vi "inputs_to_commands.vi"(11 "Joysticks":T6) -> (3 "Commands":T1)   [LabVIEW 2012]
uses:
  <vilib>/Rock Robotics/WPI/Joystick/WPI_JoystickButtonState.ctl
  Commands.ctl
  mecanum/mecanum_control.ctl
  Shooter/shooter_cmds.ctl
  climber/climber_cmds.ctl
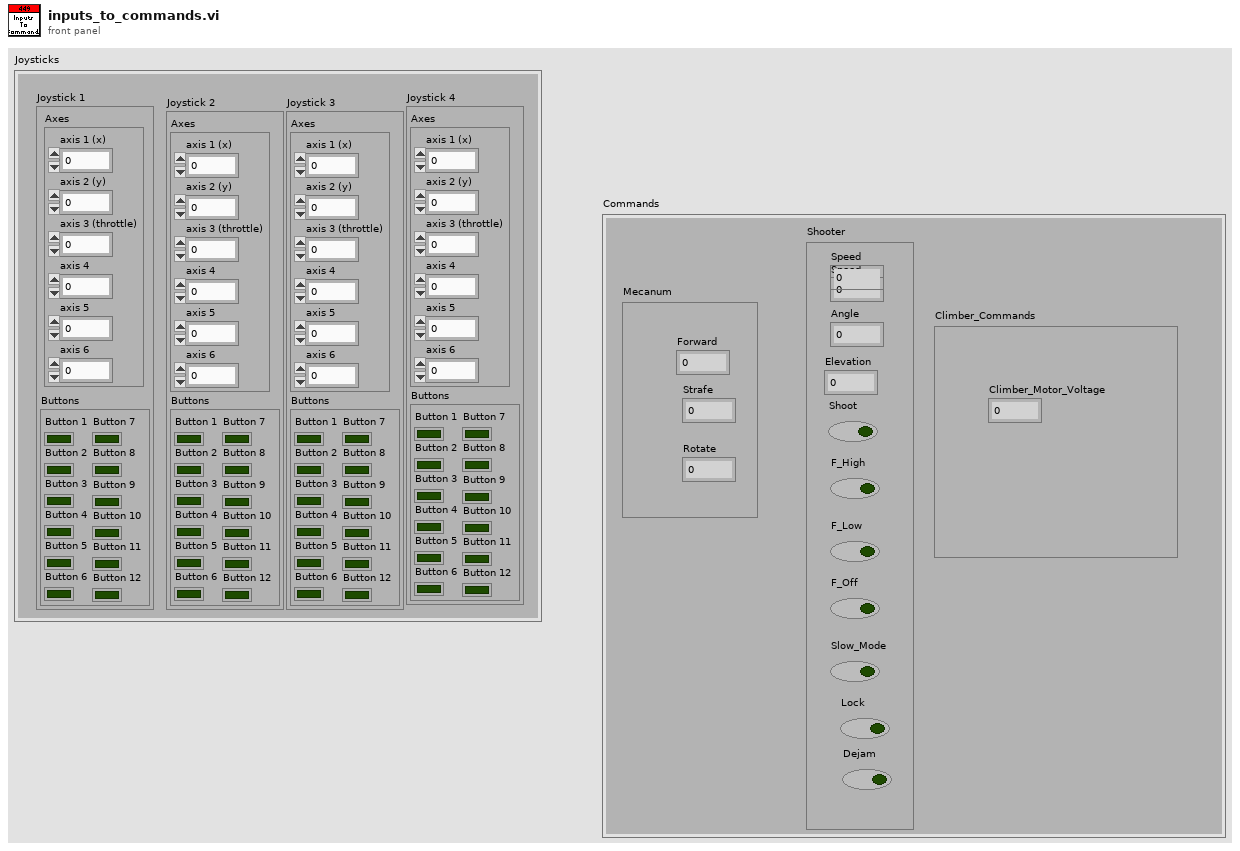
[diagram p1: front panel]
types:
  T1 = typedef "Commands.ctl" = cluster{"Mecanum":T2, "Shooter":T3, "Climber_Commands":T4, "Speed":dbl}
  T2 = typedef "mecanum_control.ctl" = cluster{"Forward":dbl, "Strafe":dbl, "Rotate":dbl}
  T3 = typedef "shooter_cmds.ctl" = cluster{"Elevation":dbl, "Shoot":bool, "F_High":bool, "F_Low":bool, "F_Off":bool, "Slow_Mode":bool, "Lock":bool, "Dejam":bool, "Angle":dbl, "Speed":dbl}
  T4 = typedef "climber_cmds.ctl" = cluster{"Climber_Motor_Voltage":dbl}
  T5 = typedef "WPI_JoystickButtonState.ctl" = cluster{"Button 1":bool, "Button 2":bool, "Button 3":bool, "Button 4":bool, "Button 5":bool, "Button 6":bool, "Button 7":bool, "Button 8":bool, "Button 9":bool, "Button 10":bool, "Button 11":bool, "Button 12":bool}
  T6 = cluster{"Joystick 1":cluster{"Axes":cluster{"axis 1 (x)":dbl, "axis 2 (y)":dbl, "axis 3 (throttle)":dbl, "axis 4":dbl, "axis 5":dbl, "axis 6":dbl}, "Buttons":T5}, "Joystick 2":cluster{"Axes":cluster{"axis 1 (x)":dbl, "axis 2 (y)":dbl, "axis 3 (throttle)":dbl, "axis 4":dbl, "axis 5":dbl, "axis 6":dbl}, "Buttons":T5}, "Joystick 3":cluster{"Axes":cluster{"axis 1 (x)":dbl, "axis 2 (y)":dbl, "axis 3 (throttle)":dbl, "axis 4":dbl, "axis 5":dbl, "axis 6":dbl}, "Buttons":T5}, "Joystick 4":cluster{"Axes":cluster{"axis 1 (x)":dbl, "axis 2 (y)":dbl, "axis 3 (throttle)":dbl, "axis 4":dbl, "axis 5":dbl, "axis 6":dbl}, "Buttons":T5}}
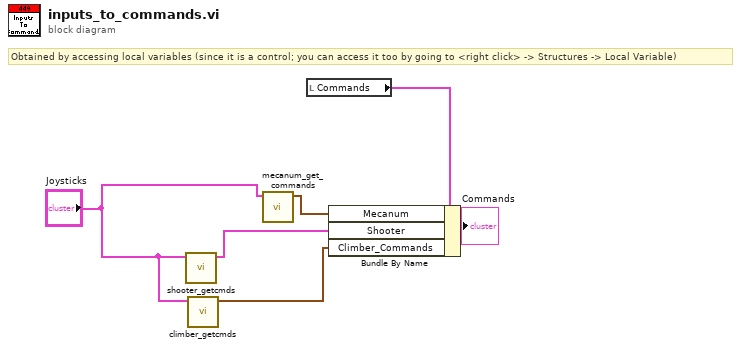
[diagram p0: block diagram]
diagram:
  # "Obtained by accessing local variables (since it is a control; you can access it too by going to <right click> -> Structures -> Local Variable)"
  n1 = call "shooter_getcmds.vi"("Joysticks"="Joysticks") -> ("Shooter"=w3:T3)  [unwired: 10 in]
  n2 = call "climber_getcmds.vi"("Joysticks"="Joysticks") -> ("Climber_Commands"=w1:T4)  [unwired: 10 in]
  n3 = call "mecanum_get_commands.vi"("Joysticks"="Joysticks") -> ("Mecanum"=w4:T2)  [unwired: 10 in]
  n4 = local read "Commands"() -> (w6:T1)
  n5 = Bundle By Name(cluster=w6, "Mecanum"=w4, "Shooter"=w3, "Climber_Commands"=w1) -> (→"Commands":T1)
